vi "Set Stage Position.vi"(3 "Position":cluster{dbl, dbl, dbl}, 4 "error in":errorcluster, 5 "VISA resource name in":refnum<visa-resource-name>) -> (1 "error out":errorcluster, 2 "VISA resource name out":refnum<visa-resource-name>)   [LabVIEW 2010]
uses:
  <vilib>/Instr/_visa.llb/VISA Configure Serial Port (Instr).vi
panel:
  out "concatenated string":string
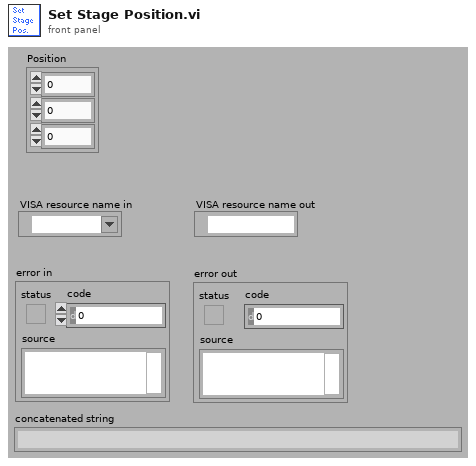
[diagram p1: front panel]
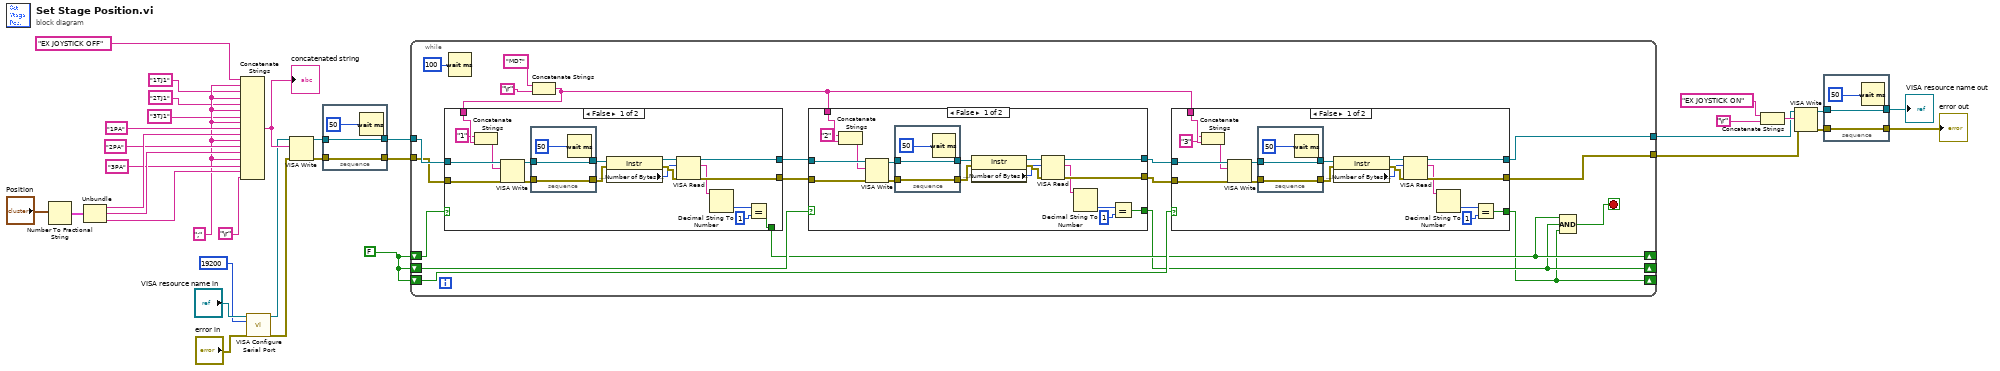
[diagram p0: block diagram]
diagram:
  w1 = FALSE
  w5 = ";"
  n1 = Number To Fractional String(number="Position") -> (F-format string=w26:cluster{string, string, string})  [unwired: 3 out]
  n2 = Unbundle(w26) -> (w25:string, w24:string, w23:string)
  n3 = Concatenate Strings("EX JOYSTICK OFF", w5, "1TJ1", w5, "2TJ1", w5, "3TJ1", w5, "1PA", w25, w5, "2PA", w24, w5, "3PA", w23, "\r") -> (w19:string)
  "concatenated string" <- w19
  n4 = call-poly "VISA Configure Serial Port"("VISA resource name"="VISA resource name in", "baud rate (9600)"=u32 19200, "error in (no error)"="error in") -> ("VISA resource name out"=w14:refnum<visa-resource-name>, "error out"=w13:errorcluster)  [unwired: 3 in, 8 out]
  n5 = VISA Write(VISA resource name=w14, write buffer=w19, error in (no error)=w13) -> (VISA resource name out=w18:refnum<visa-resource-name>, error out=w17:errorcluster)  [unwired: 1 out]
  n6 = stacked-sequence {
    tunnel: [w37] -> w29
    tunnel: w18 -> [w37]
    tunnel: w17 -> [w36]
    tunnel: [w36] -> w28
    frame #0 {
      n7 = Wait (ms)(milliseconds to wait=50) -> ()  [unwired: 1 out]
    }
  }
  n8 = while {
    tunnel: w29 -> [w56]
    tunnel: w28 -> [w55]
    tunnel: [w43] -> w7
    tunnel: [w42] -> w6
    shift-right: [w41] -> _
    shift-left: w1 -> [w51]
    shift-right: [w40] -> _
    shift-left: w1 -> [w45]
    shift-right: [w39] -> _
    shift-left: w1 -> [w44]
    stop <- w38 stop-if-true
    n9 = Wait (ms)(milliseconds to wait=u32 100) -> ()  [unwired: 1 out]
    n10 = Concatenate Strings("MD?" ("write buffer"), "\r") -> (w46:string)
    n11 = case shown="False" w51 {
      selector: w51 -> [_ w128]
      tunnel: w56 -> [w122 w126]
      tunnel: w55 -> [w121 w127]
      tunnel: [w120 w126] -> w50
      tunnel: [w119 w127] -> w49
      tunnel: w46 -> [w108 _]
      tunnel: [w105 w128] -> w41
      frame False {
        n12 = Concatenate Strings("1" ("string"), w108) -> (w106:string)
        n13 = VISA Write(VISA resource name=w122, write buffer=w106, error in (no error)=w121) -> (VISA resource name out=w110:refnum<visa-resource-name>, error out=w111:errorcluster)  [unwired: 1 out]
        n14 = stacked-sequence {
          tunnel: [w125] -> w112
          tunnel: w110 -> [w125]
          tunnel: w111 -> [w124]
          tunnel: [w124] -> w116
          frame #0 {
            n15 = Wait (ms)(milliseconds to wait=50) -> ()  [unwired: 1 out]
          }
        }
        n16 = property class="Instr"(reference=w112, error in=w116) -> (reference out=w113:refnum<visa-resource-name>, error out=w115:errorcluster, "Serial Settings:Number of Bytes at Serial Port"=w114:u32)
        n17 = VISA Read(VISA resource name=w113, byte count=w114, error in (no error)=w115) -> (VISA resource name out=w120:refnum<visa-resource-name>, read buffer=w109:string, error out=w119:errorcluster)  [unwired: 1 out]
        n18 = Decimal String To Number(string=w109) -> (number=w117:i32)  [unwired: 3 out]
        n19 = Equal?(x=w117, y=1) -> (x = y?=w105:bool)
      }
      frame True {
      }
    }
    n20 = case shown="False" w45 {
      selector: w45 -> [_ w104]
      tunnel: w50 -> [w98 w102]
      tunnel: w49 -> [w97 w103]
      tunnel: [w96 w102] -> w48
      tunnel: [w95 w103] -> w47
      tunnel: w46 -> [w84 _]
      tunnel: [w81 w104] -> w40
      frame False {
        n21 = Concatenate Strings("2" ("string"), w84) -> (w82:string)
        n22 = VISA Write(VISA resource name=w98, write buffer=w82, error in (no error)=w97) -> (VISA resource name out=w86:refnum<visa-resource-name>, error out=w87:errorcluster)  [unwired: 1 out]
        n23 = stacked-sequence {
          tunnel: [w101] -> w88
          tunnel: w86 -> [w101]
          tunnel: w87 -> [w100]
          tunnel: [w100] -> w92
          frame #0 {
            n24 = Wait (ms)(milliseconds to wait=50) -> ()  [unwired: 1 out]
          }
        }
        n25 = property class="Instr"(reference=w88, error in=w92) -> (reference out=w89:refnum<visa-resource-name>, error out=w91:errorcluster, "Serial Settings:Number of Bytes at Serial Port"=w90:u32)
        n26 = VISA Read(VISA resource name=w89, byte count=w90, error in (no error)=w91) -> (VISA resource name out=w96:refnum<visa-resource-name>, read buffer=w85:string, error out=w95:errorcluster)  [unwired: 1 out]
        n27 = Decimal String To Number(string=w85) -> (number=w93:i32)  [unwired: 3 out]
        n28 = Equal?(x=w93, y=1) -> (x = y?=w81:bool)
      }
      frame True {
      }
    }
    n29 = case shown="False" w44 {
      selector: w44 -> [_ w80]
      tunnel: w48 -> [w74 w78]
      tunnel: w47 -> [w73 w79]
      tunnel: [w72 w78] -> w43
      tunnel: [w71 w79] -> w42
      tunnel: w46 -> [w60 _]
      tunnel: [w57 w80] -> w39
      frame False {
        n30 = Concatenate Strings("3" ("string"), w60) -> (w58:string)
        n31 = VISA Write(VISA resource name=w74, write buffer=w58, error in (no error)=w73) -> (VISA resource name out=w62:refnum<visa-resource-name>, error out=w63:errorcluster)  [unwired: 1 out]
        n32 = stacked-sequence {
          tunnel: [w77] -> w64
          tunnel: w62 -> [w77]
          tunnel: w63 -> [w76]
          tunnel: [w76] -> w68
          frame #0 {
            n33 = Wait (ms)(milliseconds to wait=50) -> ()  [unwired: 1 out]
          }
        }
        n34 = property class="Instr"(reference=w64, error in=w68) -> (reference out=w65:refnum<visa-resource-name>, error out=w67:errorcluster, "Serial Settings:Number of Bytes at Serial Port"=w66:u32)
        n35 = VISA Read(VISA resource name=w65, byte count=w66, error in (no error)=w67) -> (VISA resource name out=w72:refnum<visa-resource-name>, read buffer=w61:string, error out=w71:errorcluster)  [unwired: 1 out]
        n36 = Decimal String To Number(string=w61) -> (number=w69:i32)  [unwired: 3 out]
        n37 = Equal?(x=w69, y=1) -> (x = y?=w57:bool)
      }
      frame True {
      }
    }
    n38 = Compound Arithmetic op=AND(w41, w40, w39) -> (w38:bool)
  }
  n39 = Concatenate Strings("EX JOYSTICK ON" ("write buffer"), "\r") -> (w12:string)
  n40 = VISA Write(VISA resource name=w7, write buffer=w12, error in (no error)=w6) -> (VISA resource name out=w9:refnum<visa-resource-name>, error out=w10:errorcluster)  [unwired: 1 out]
  n41 = stacked-sequence {
    tunnel: [w131] -> w31
    tunnel: w9 -> [w131]
    tunnel: w10 -> [w130]
    tunnel: [w130] -> w30
    frame #0 {
      n42 = Wait (ms)(milliseconds to wait=50) -> ()  [unwired: 1 out]
    }
  }
  "VISA resource name out" <- w31
  "error out" <- w30
